vi "test CAN Cyclic Loopback with Disable Channels.vi"(8 "error in (no error)":errorcluster, 11 "TestCase in":refnum<class "CAN Loopback Tests.lvclass">) -> (0 "error out":errorcluster, 3 "TestCase out":refnum<class "CAN Loopback Tests.lvclass">)   [LabVIEW 2017, in "CAN Loopback Tests.lvclass"]
uses:
  CAN Loopback Tests.lvclass
  <vilib>/addons/_JKI Toolkits/VI Tester/TestCase.llb/TestCase.lvclass
  C:/Program Files (x86)/National Instruments/LabVIEW 2017/vi.lib/addons/_JKI Toolkits/VI Tester/TestCase.llb/TestCase.lvclass
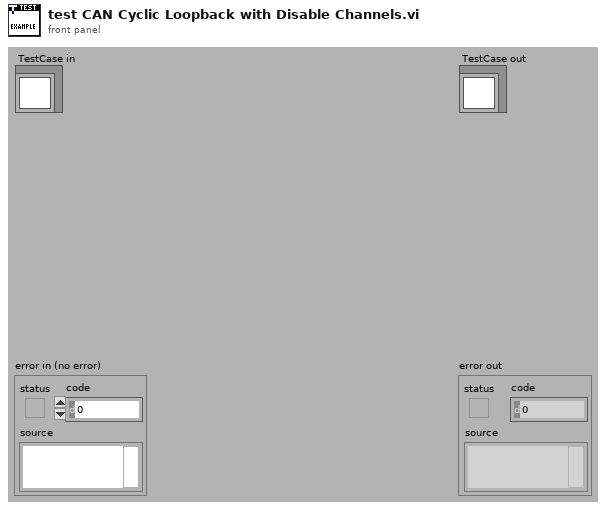
[diagram p1: front panel]
types:
  T1 = cluster{"loopback channels to write":string[], "loopback channels to read":string[], "additional channels to write":string[], "additional channels to read":string[]}
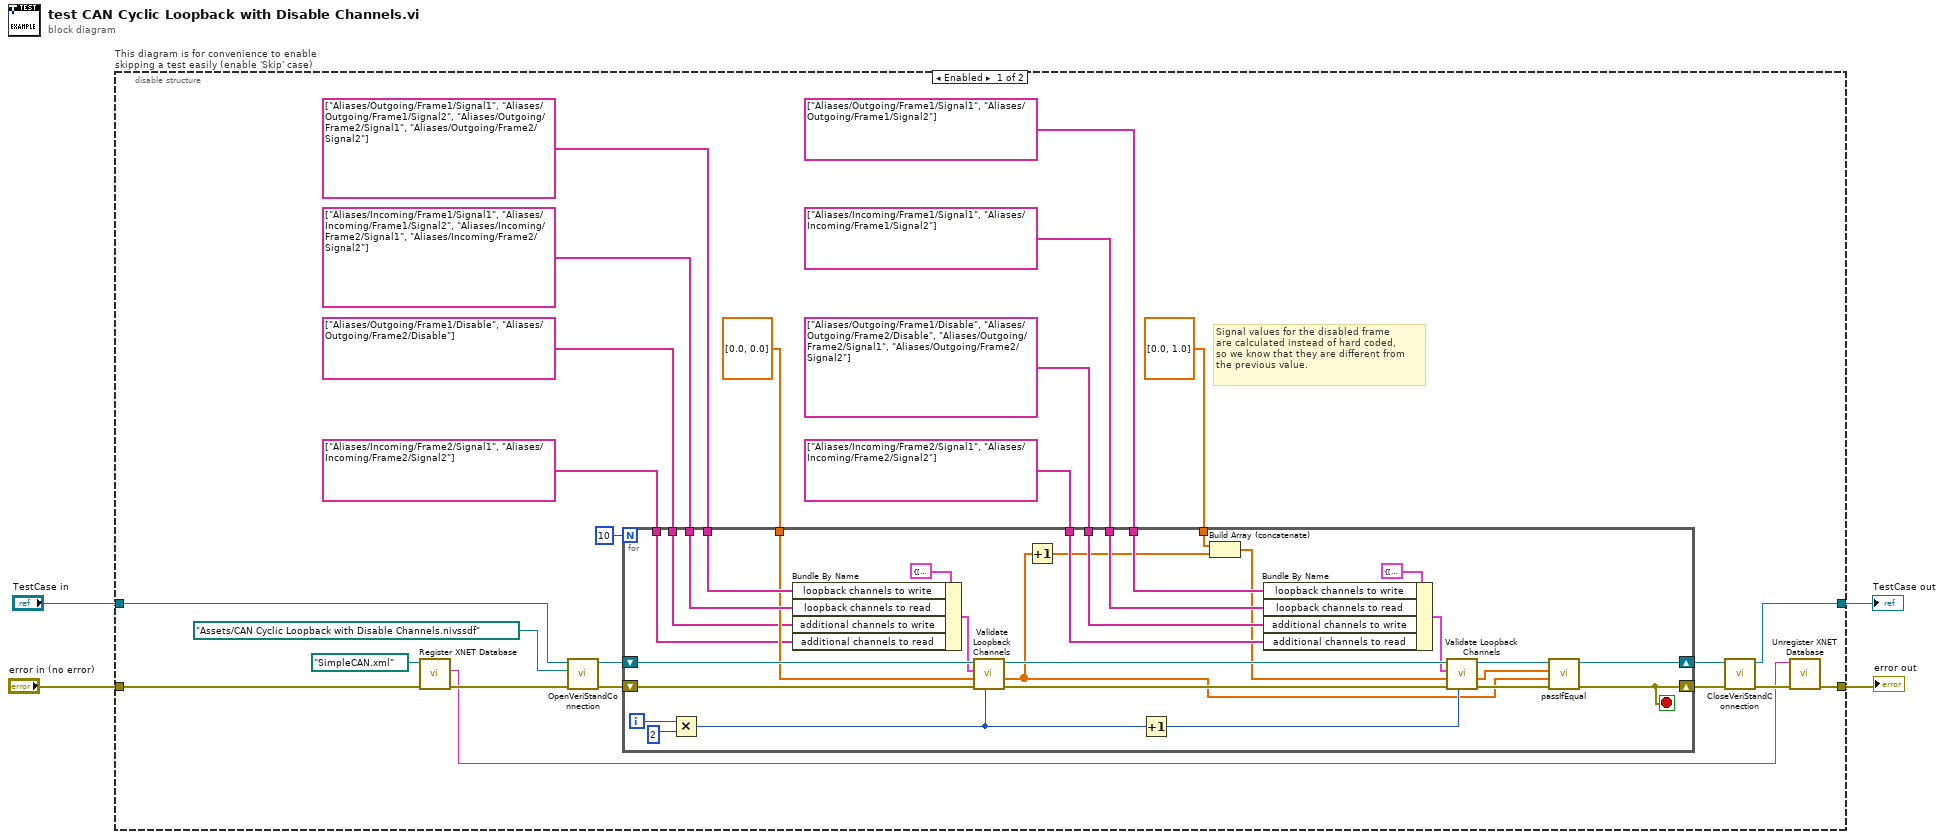
[diagram p0: block diagram]
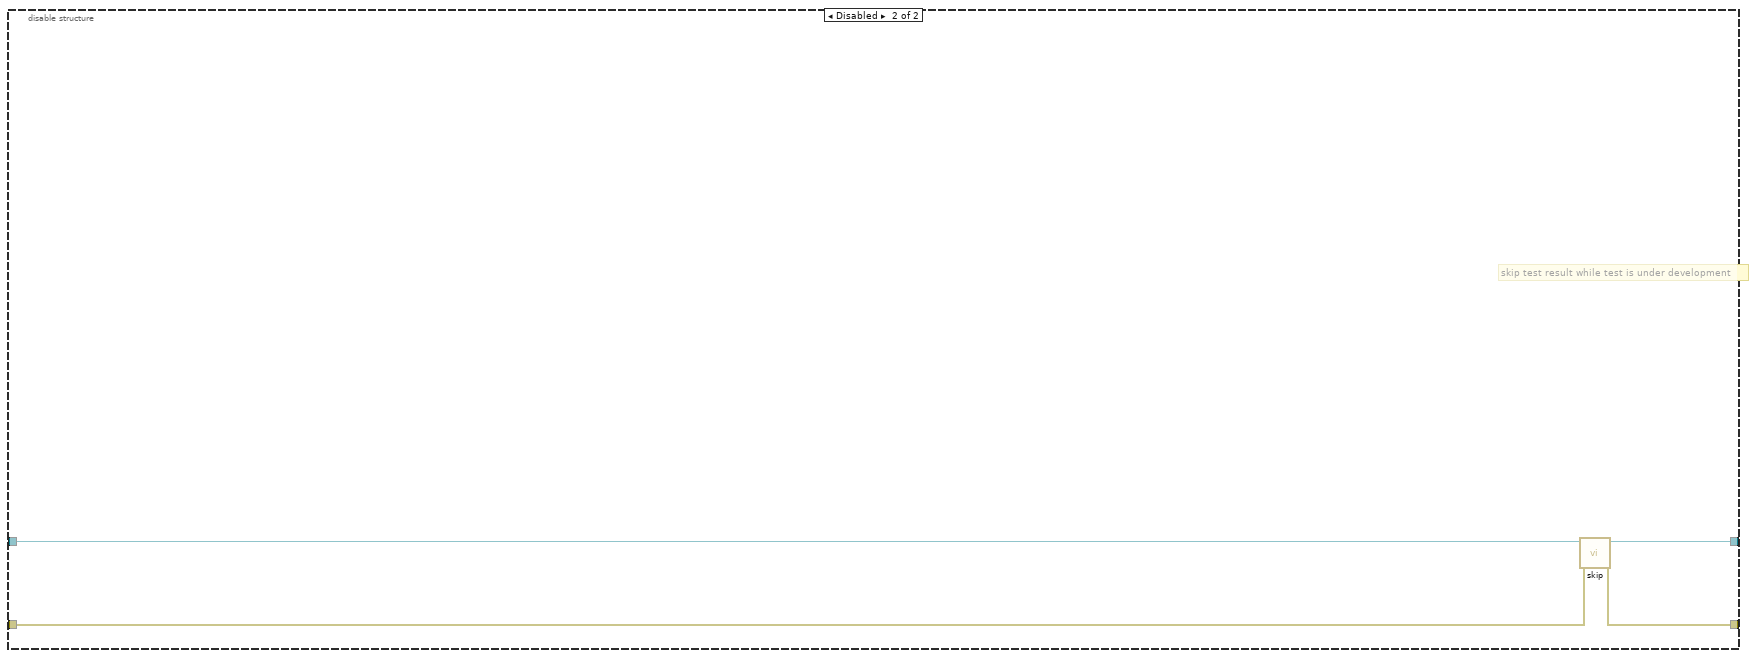
[diagram p2: hidden frame]
diagram:
  n1 = disable-structure "This diagram is for convenience to enable skipping a test easily (enable 'Skip' case)" shown="Enabled" {
    disable-tunnel: "TestCase in" -> [w28 w62]
    disable-tunnel: [w26 w60] -> w1
    disable-tunnel: [w17 w61] -> w3
    disable-tunnel: "error in (no error)" -> [w19 w59]
    frame Enabled {
      # "Signal values for the disabled frame\nare calculated instead of hard coded,\nso we know that they are different from\nthe previous value."
      n2 = call "Register XNET Database.vi"("error in (no error)"=w19, "database path"=path "SimpleCAN.xml") -> ("error out"=w18:errorcluster, "alias"=w15:string)  [unwired: 8 in]
      n3 = call-dynamic "OpenVeriStandConnection.vi"("error in (no error)"=w18, "System Definition File"=path "Assets/CAN Cyclic Loopback with Disable Channels.nivssdf", "VeriStand Test Case in"=w28) -> ("error out"=w12:errorcluster, "VeriStand Test Case out"=w10:refnum<class "CAN Loopback Tests.lvclass">)  [unwired: 6 in, 1 out]
      n4 = for {
        N: 10 -> [_]
        shift-right: [w36] -> w24
        shift-left: w12 -> [w58]
        shift-right: [w34] -> w25
        shift-left: w10 -> [w57]
        tunnel: string[] ["Aliases/Incoming/Frame1/Signal1", "Aliases/Incoming/Frame1/Signal2", "Aliases/Incoming/Frame2/Signal1", "Aliases/Incoming/Frame2/Signal2"] -> [w55]
        tunnel: string[] ["Aliases/Outgoing/Frame1/Signal1", "Aliases/Outgoing/Frame1/Signal2", "Aliases/Outgoing/Frame2/Signal1", "Aliases/Outgoing/Frame2/Signal2"] -> [w56]
        tunnel: string[] ["Aliases/Outgoing/Frame1/Disable", "Aliases/Outgoing/Frame2/Disable"] -> [w49]
        tunnel: dbl[] [0.0, 0.0] ("additional channel values to write") -> [w52]
        tunnel: dbl[] [0.0, 1.0] ("additional channel values to write") -> [w31]
        tunnel: string[] ["Aliases/Outgoing/Frame1/Disable", "Aliases/Outgoing/Frame2/Disable", "Aliases/Outgoing/Frame2/Signal1", "Aliases/Outgoing/Frame2/Signal2"] -> [w41]
        tunnel: string[] ["Aliases/Incoming/Frame1/Signal1", "Aliases/Incoming/Frame1/Signal2"] -> [w40]
        tunnel: string[] ["Aliases/Outgoing/Frame1/Signal1", "Aliases/Outgoing/Frame1/Signal2"] -> [w39]
        tunnel: string[] ["Aliases/Incoming/Frame2/Signal1", "Aliases/Incoming/Frame2/Signal2"] -> [w38]
        tunnel: string[] ["Aliases/Incoming/Frame2/Signal1", "Aliases/Incoming/Frame2/Signal2"] -> [w37]
        i -> [w51]
        stop <- w36 stop-if-true
        n5 = Multiply(x=w51, y=2) -> (x*y=w45:i32)
        n6 = Bundle By Name(cluster=T1 {"loopback channels to write"=[], "loopback channels to read"=[], "additional channels to write"=[], "additional channels to read"=[]} ("channels"), "loopback channels to write"=w56, "loopback channels to read"=w55, "additional channels to write"=w49, "additional channels to read"=w37) -> (w53:T1)
        n7 = call "Validate Loopback Channels.vi"("index"=w45, "error in (no error)"=w58, "additional channel values to write"=w52, "channels"=w53, "CAN Loopback Tests in"=w57) -> ("error out"=w48:errorcluster, "additional channel values to read"=w32:dbl[], "CAN Loopback Tests out"=w47:refnum<class "CAN Loopback Tests.lvclass">)  [unwired: 3 in, 1 out]
        n8 = Increment(x=w32) -> (x+1=w30:dbl[])
        n9 = Increment(x=w45) -> (x+1=w44:i32)
        n10 = Build Array (concatenate)(w31, w30) -> (w29:dbl[])
        n11 = Bundle By Name(cluster=T1 {"loopback channels to write"=[], "loopback channels to read"=[], "additional channels to write"=[], "additional channels to read"=[]} ("channels"), "loopback channels to write"=w39, "loopback channels to read"=w40, "additional channels to write"=w41, "additional channels to read"=w38) -> (w42:T1)
        n12 = call "Validate Loopback Channels.vi"("index"=w44, "error in (no error)"=w48, "additional channel values to write"=w29, "channels"=w42, "CAN Loopback Tests in"=w47) -> ("error out"=w46:errorcluster, "additional channel values to read"=w33:dbl[], "CAN Loopback Tests out"=w35:refnum<class "CAN Loopback Tests.lvclass">)  [unwired: 3 in, 1 out]
        n13 = call-dynamic "passIfEqual.vi"("error in (no error)"=w46, "y"=w32, "x"=w33, "TestCase in"=w35) -> ("error out"=w36:errorcluster, "TestCase out"=w34:refnum<class "CAN Loopback Tests.lvclass">)  [unwired: 6 in]
      }
      n14 = call-dynamic "CloseVeriStandConnection.vi"("error in (no error)"=w24, "VeriStand Test Case in"=w25) -> ("error out"=w16:errorcluster, "VeriStand Test Case out"=w26:refnum<class "CAN Loopback Tests.lvclass">)  [unwired: 8 in]
      n15 = call "Unregister XNET Database.vi"("error in (no error)"=w16, "alias"=w15) -> ("error out"=w17:errorcluster)  [unwired: 9 in]
    }
    frame Disabled {
      # "skip test result while test is under development"
      n16 = call <vilib>:"skip.vi"("error in (no error)"=w59, "TestCase in"=w62) -> ("error out"=w61:errorcluster, "TestCase out"=w60:refnum<class "CAN Loopback Tests.lvclass">)  [unwired: 8 in]
    }
  }
  "error out" <- w3
  "TestCase out" <- w1
